vi "PID (SubVI).vi"(0 "Feedback":i32, 1 "K":dbl, 2 "Reference":dbl, 3 "I":dbl, 4 "D":dbl) -> (5 "Control Out":dbl)   [LabVIEW 2010]
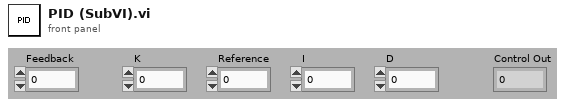
[diagram p1: front panel]
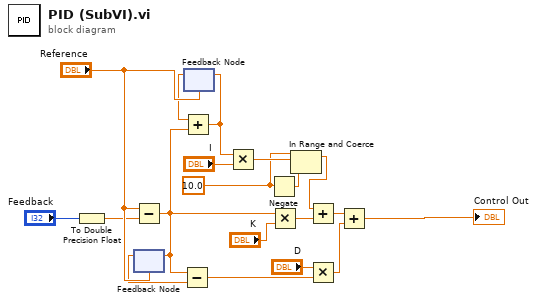
[diagram p0: block diagram]
diagram:
  w3 = 10.0 ("Max")
  n1 = To Double Precision Float(number="Feedback") -> (double precision float=w5:dbl)
  n2 = Subtract(x="Reference", y=w5) -> (x-y=w17:dbl)
  n3 = feedback-in #1(w17) -> ()
  n4 = feedback #1("Reference") -> (w12:dbl)
  n5 = Subtract(x=w17, y=w12) -> (x-y=w7:dbl)
  n6 = feedback #2("Reference") -> (w13:dbl)
  n7 = Add(x=w13, y=w17) -> (x+y=w14:dbl)
  n8 = feedback-in #2(w14) -> ()
  n9 = Multiply(x=w14, y="I") -> (x*y=w4:dbl)
  n10 = Negate(x=w3) -> (-x=w2:dbl)
  n11 = Multiply(x=w17, y="K") -> (x*y=w11:dbl)
  n12 = In Range and Coerce(upper limit=w3, x=w4, lower limit=w2) -> (coerced(x)=w1:dbl)  [unwired: 1 out]
  n13 = Add(x=w1, y=w11) -> (x+y=w10:dbl)
  n14 = Multiply(x="D", y=w7) -> (x*y=w9:dbl)
  n15 = Add(x=w10, y=w9) -> (x+y=→"Control Out":dbl)
